vi "PrototypeV2_control.vi"() -> ()   [LabVIEW 2019]
uses:
  <vilib>/Instr/_visa.llb/VISA Configure Serial Port (Instr).vi
panel:
  out "CONV2":cluster{dbl, dbl, dbl}(graph)
  out "converter2 file":path
  out "controller file":path
  out "converter1 file":path
  in  "CONVERTER 2 PORT":refnum<visa-resource-name>="COM4"
  out "sync":bool
  in  "CONVERTER 2":bool
  in  "CONVERTER 1 PORT":refnum<visa-resource-name>="COM4"
  out "sync":bool
  in  "CONVERTER 1":bool
  out "CONV1":cluster{dbl, dbl, dbl}(graph)
  out "3.3V REG":cluster{dbl, dbl}(graph)
  out "5V REG":cluster{dbl, dbl}(graph)
  out "BUS":cluster{dbl, dbl, dbl}(graph)
  in  "project name":string
  in  "START":bool
  in  "CONTROLLER PORT":refnum<visa-resource-name>="COM4"
  out "sync":bool
  in  "CONTROLLER":bool
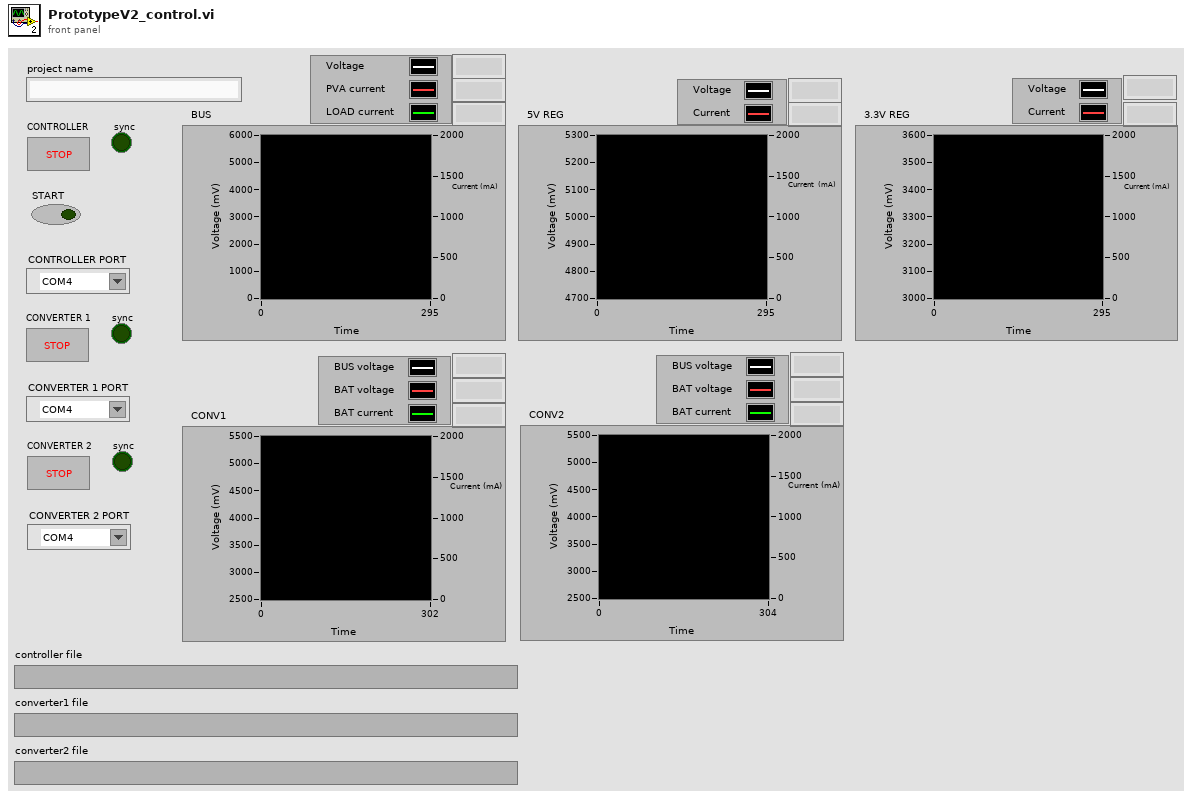
[diagram p1: front panel]
types:
  T1 = cluster{u16, u16, u16, u16, u16, u16, u16, u16, u16}
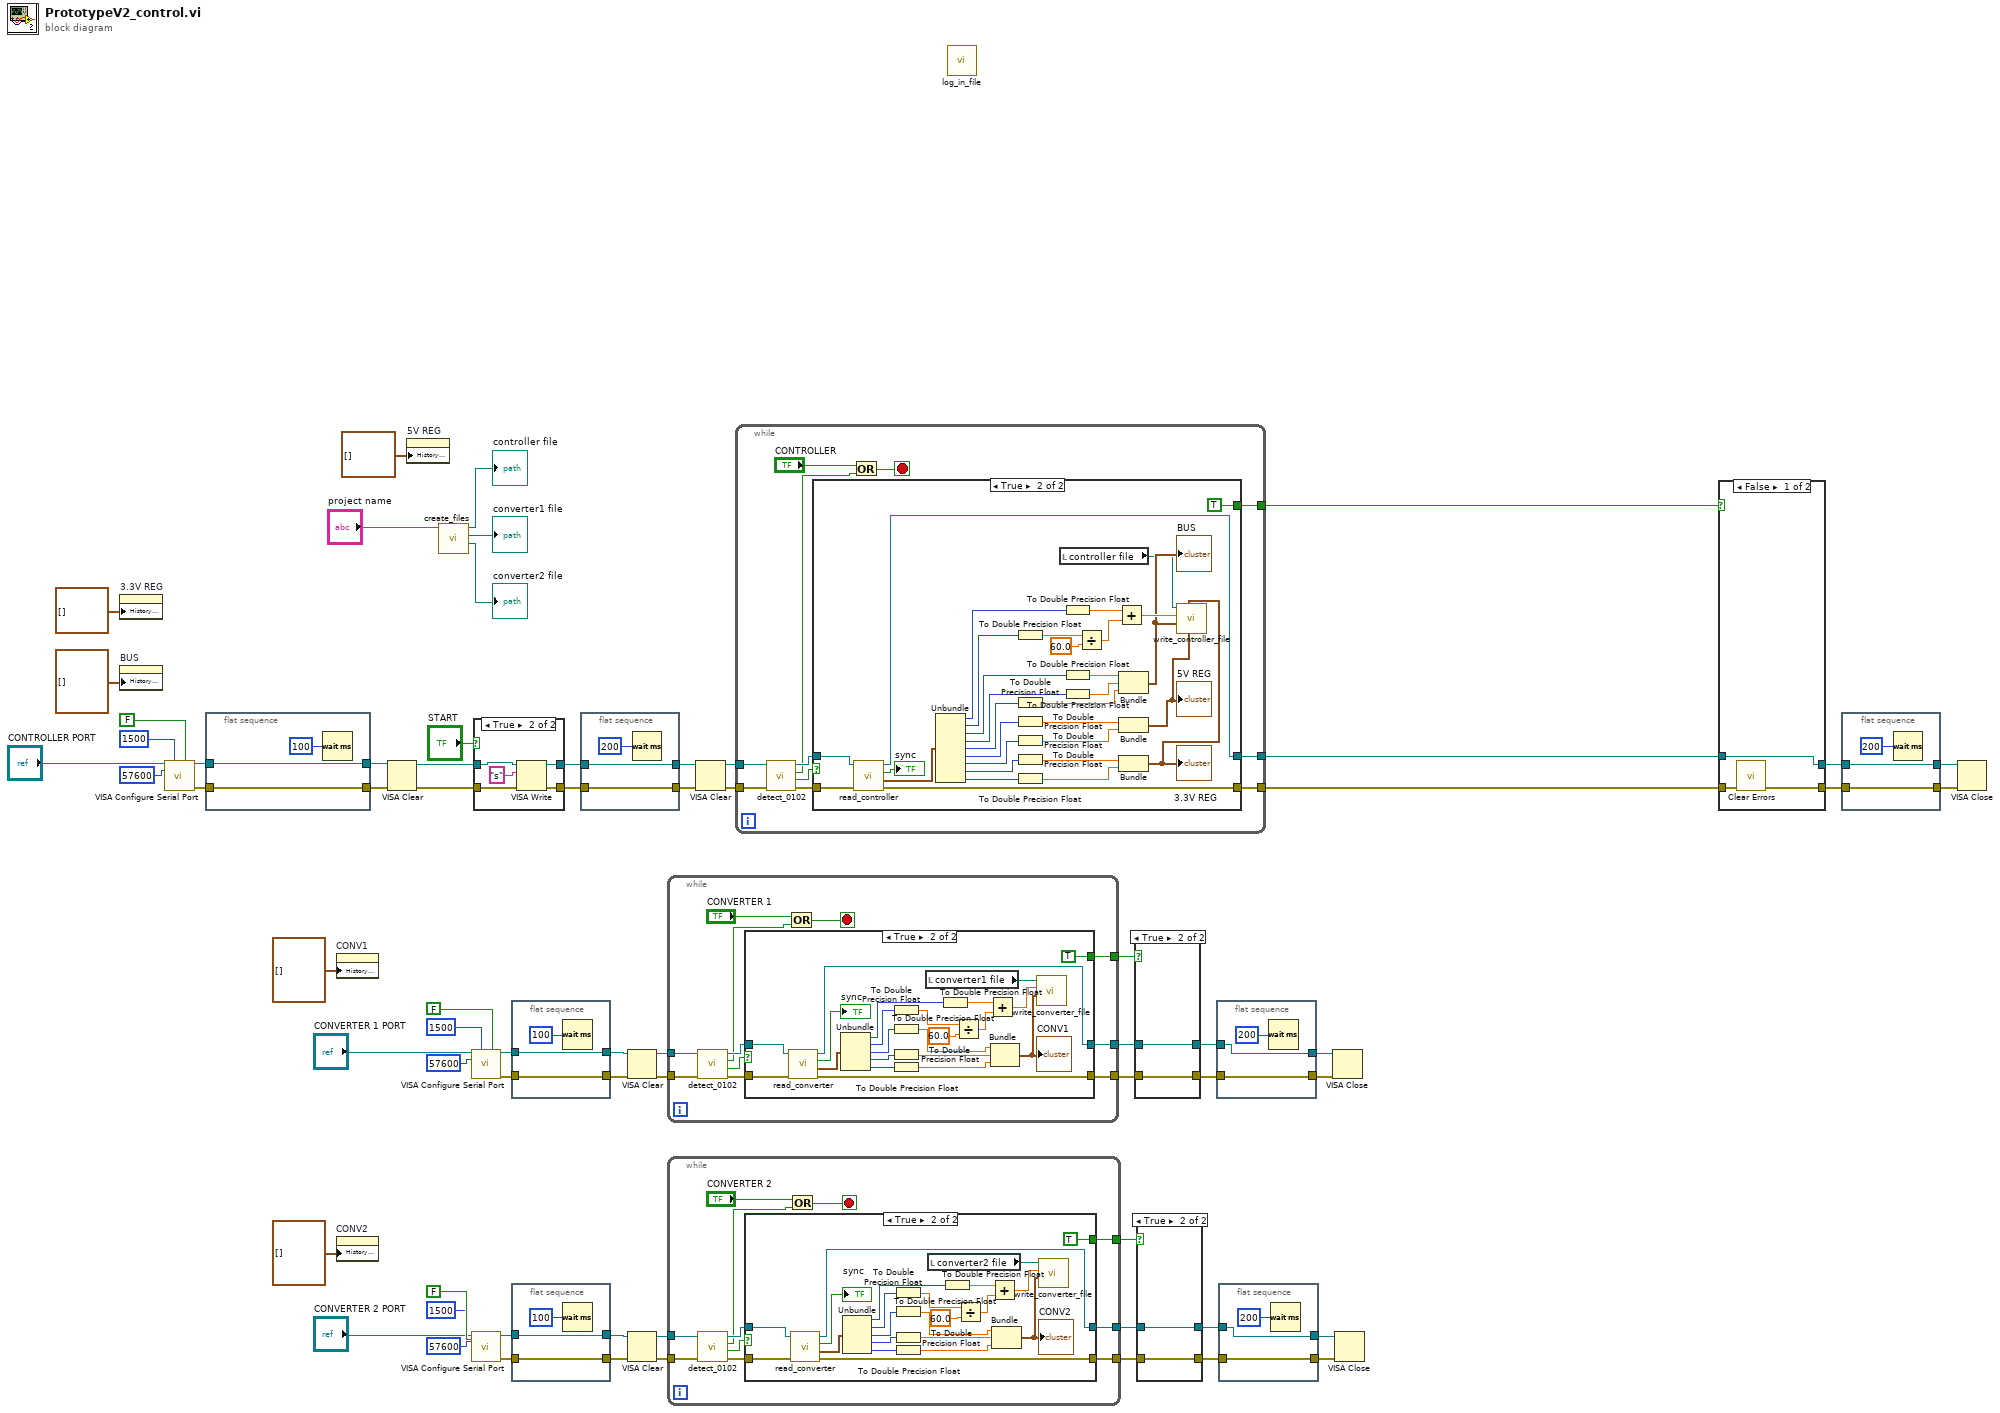
[diagram p0: block diagram]
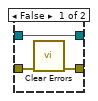
[diagram p2: hidden frame]
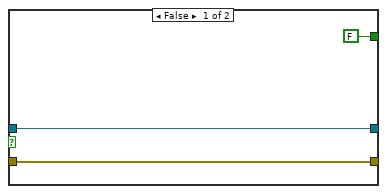
[diagram p3: hidden frame]
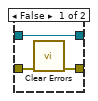
[diagram p4: hidden frame]
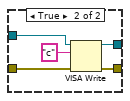
[diagram p5: hidden frame]
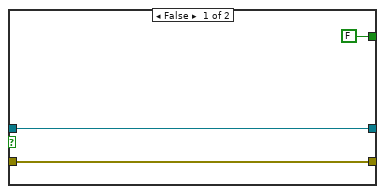
[diagram p6: hidden frame]
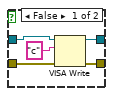
[diagram p7: hidden frame]
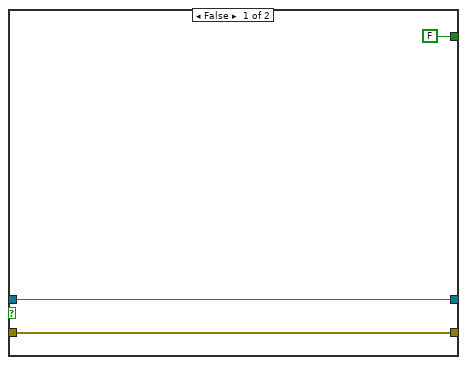
[diagram p8: hidden frame]
diagram:
  n1 = property on="3.3V REG" class="WFChart (strict)"("History Data"=cluster{dbl, dbl}[] []) -> ()  [unwired: 2 in, 2 out]
  n2 = property on="BUS" class="WFChart (strict)"("History Data"=cluster{dbl, dbl, dbl}[] []) -> ()  [unwired: 2 in, 2 out]
  n3 = call-poly "VISA Configure Serial Port"("VISA resource name"="CONTROLLER PORT", "timeout (10sec)"=u32 1500, "Enable Termination\nChar (T)"=FALSE ("Enable Termination\nChar (T)"), "baud rate (9600)"=u32 57600) -> ("VISA resource name out"=w64:refnum<visa-resource-name>, "error out"=w63:errorcluster)  [unwired: 10 in]
  n4 = flat-sequence {
    tunnel: w63 -> [w69]
    tunnel: [w69] -> w62
    tunnel: [w68] -> w61
    tunnel: w64 -> [w68]
    frame #0 {
      n5 = Wait (ms)(milliseconds to wait=u32 100) -> ()  [unwired: 1 out]
    }
  }
  n6 = property on="CONV1" class="WFChart (strict)"("History Data"=cluster{dbl, dbl, dbl}[] []) -> ()  [unwired: 2 in, 2 out]
  n7 = property on="CONV2" class="WFChart (strict)"("History Data"=cluster{dbl, dbl, dbl}[] []) -> ()  [unwired: 2 in, 2 out]
  n8 = VISA Clear(VISA resource name=w61, error in (no error)=w62) -> (VISA resource name out=w60:refnum<visa-resource-name>, error out=w59:errorcluster)
  n9 = property on="5V REG" class="WFChart (strict)"("History Data"=cluster{dbl, dbl}[] []) -> ()  [unwired: 2 in, 2 out]
  n10 = call "create_files.vi"("project name"="project name") -> ("converter2"=→"converter2 file":path, "converter1"=→"converter1 file":path, "controller"=→"controller file":path)  [unwired: 8 in]
  n11 = call-poly "VISA Configure Serial Port"("VISA resource name"="CONVERTER 1 PORT", "timeout (10sec)"=u32 1500, "Enable Termination\nChar (T)"=FALSE ("Enable Termination\nChar (T)"), "baud rate (9600)"=u32 57600) -> ("VISA resource name out"=w39:refnum<visa-resource-name>, "error out"=w38:errorcluster)  [unwired: 10 in]
  n12 = call-poly "VISA Configure Serial Port"("VISA resource name"="CONVERTER 2 PORT", "timeout (10sec)"=u32 1500, "Enable Termination\nChar (T)"=FALSE ("Enable Termination\nChar (T)"), "baud rate (9600)"=u32 57600) -> ("VISA resource name out"=w16:refnum<visa-resource-name>, "error out"=w15:errorcluster)  [unwired: 10 in]
  n13 = case shown="True" "START" {
    tunnel: w60 -> [w74 w80]
    tunnel: [w72 w79] -> w57
    tunnel: w59 -> [w73 w78]
    tunnel: [w71 w77] -> w56
    frame False {
      n14 = VISA Write(VISA resource name=w74, write buffer="c", error in (no error)=w73) -> (VISA resource name out=w72:refnum<visa-resource-name>, error out=w71:errorcluster)  [unwired: 1 out]
    }
    frame True {
      n15 = VISA Write(VISA resource name=w80, write buffer="s", error in (no error)=w78) -> (VISA resource name out=w79:refnum<visa-resource-name>, error out=w77:errorcluster)  [unwired: 1 out]
    }
  }
  n16 = flat-sequence {
    tunnel: w38 -> [w82]
    tunnel: [w82] -> w37
    tunnel: [w81] -> w36
    tunnel: w39 -> [w81]
    frame #0 {
      n17 = Wait (ms)(milliseconds to wait=u32 100) -> ()  [unwired: 1 out]
    }
  }
  n18 = flat-sequence {
    tunnel: w15 -> [w85]
    tunnel: [w85] -> w14
    tunnel: [w84] -> w13
    tunnel: w16 -> [w84]
    frame #0 {
      n19 = Wait (ms)(milliseconds to wait=u32 100) -> ()  [unwired: 1 out]
    }
  }
  n20 = flat-sequence {
    tunnel: w56 -> [w88]
    tunnel: [w88] -> w53
    tunnel: [w87] -> w55
    tunnel: w57 -> [w87]
    frame #0 {
      n21 = Wait (ms)(milliseconds to wait=u32 200) -> ()  [unwired: 1 out]
    }
  }
  n22 = VISA Clear(VISA resource name=w36, error in (no error)=w37) -> (VISA resource name out=w21:refnum<visa-resource-name>, error out=w20:errorcluster)
  n23 = VISA Clear(VISA resource name=w13, error in (no error)=w14) -> (VISA resource name out=w4:refnum<visa-resource-name>, error out=w3:errorcluster)
  n24 = while {
    tunnel: w20 -> [w94]
    tunnel: [w99] -> w27
    tunnel: [w100] -> w28
    tunnel: w21 -> [w95]
    tunnel: [w96] -> w26
    stop <- w97 stop-if-true
    n25 = call "detect_0102.vi"("error in (no error)"=w94, "VISA Refnum in"=w95) -> ("error out"=w92:errorcluster, "RECEIVED"=w90:bool, "NOT RECEIVED"=w91:bool, "VISA Refnum out"=w93:refnum<visa-resource-name>)  [unwired: 6 in]
    n26 = case shown="True" w90 {
      tunnel: w93 -> [w103 w112]
      tunnel: w92 -> [w102 w107]
      tunnel: [w103 w108] -> w100
      tunnel: [w102 w111] -> w99
      tunnel: [FALSE TRUE] -> w96
      frame False {
      }
      frame True {
        n27 = call "read_converter.vi"("error in (no error)"=w107, "VISA Refnum in"=w112) -> ("error out"=w111:errorcluster, "Types?"=w109:cluster{u16, u16, u16, u16, i16}, "sync"=→"sync":bool, "VISA Refnum out"=w108:refnum<visa-resource-name>)  [unwired: 6 in]
        n28 = Unbundle(w109) -> (w125:u16, w124:u16, w119:u16, w118:u16, w117:i16)
        n29 = To Double Precision Float(number=w124) -> (double precision float=w122:dbl)
        n30 = To Double Precision Float(number=w119) -> (double precision float=w116:dbl)
        n31 = To Double Precision Float(number=w118) -> (double precision float=w115:dbl)
        n32 = To Double Precision Float(number=w117) -> (double precision float=w114:dbl)
        n33 = local read "converter1 file"() -> (w105:path)
        n34 = To Double Precision Float(number=w125) -> (double precision float=w121:dbl)
        n35 = Divide(x=w122, y=60.0) -> (x/y=w120:dbl)
        n36 = Add(x=w121, y=w120) -> (x+y=w106:dbl)
        n37 = Bundle(w116, w115, w114) -> (w104:cluster{dbl, dbl, dbl})  [unwired: 1 in]
        "CONV1" <- w104
        n38 = call "write_converter_file.vi"("CONVERTER"=w104, "minutes"=w106, "converter file"=w105) -> ()  [unwired: 9 in]
      }
    }
    n39 = Or(x="CONVERTER 1", y=w91) -> (x .or. y?=w97:bool)
  }
  n40 = while {
    tunnel: w3 -> [w131]
    tunnel: [w135] -> w6
    tunnel: [w136] -> w7
    tunnel: w4 -> [w132]
    tunnel: [w133] -> w5
    stop <- w134 stop-if-true
    n41 = call "detect_0102.vi"("error in (no error)"=w131, "VISA Refnum in"=w132) -> ("error out"=w129:errorcluster, "RECEIVED"=w127:bool, "NOT RECEIVED"=w128:bool, "VISA Refnum out"=w130:refnum<visa-resource-name>)  [unwired: 6 in]
    n42 = case shown="True" w127 {
      tunnel: w130 -> [w139 w148]
      tunnel: w129 -> [w138 w144]
      tunnel: [w139 w145] -> w136
      tunnel: [w138 w147] -> w135
      tunnel: [FALSE TRUE] -> w133
      frame False {
      }
      frame True {
        n43 = call "read_converter.vi"("error in (no error)"=w144, "VISA Refnum in"=w148) -> ("error out"=w147:errorcluster, "Types?"=w146:cluster{u16, u16, u16, u16, i16}, "sync"=→"sync":bool, "VISA Refnum out"=w145:refnum<visa-resource-name>)  [unwired: 6 in]
        n44 = Unbundle(w146) -> (w161:u16, w160:u16, w155:u16, w154:u16, w153:i16)
        n45 = To Double Precision Float(number=w160) -> (double precision float=w158:dbl)
        n46 = To Double Precision Float(number=w155) -> (double precision float=w152:dbl)
        n47 = To Double Precision Float(number=w154) -> (double precision float=w151:dbl)
        n48 = To Double Precision Float(number=w153) -> (double precision float=w150:dbl)
        n49 = local read "converter2 file"() -> (w140:path)
        n50 = To Double Precision Float(number=w161) -> (double precision float=w157:dbl)
        n51 = Divide(x=w158, y=60.0) -> (x/y=w156:dbl)
        n52 = Add(x=w157, y=w156) -> (x+y=w141:dbl)
        n53 = Bundle(w152, w151, w150) -> (w142:cluster{dbl, dbl, dbl})  [unwired: 1 in]
        "CONV2" <- w142
        n54 = call "write_converter_file.vi"("CONVERTER"=w142, "minutes"=w141, "converter file"=w140) -> ()  [unwired: 9 in]
      }
    }
    n55 = Or(x="CONVERTER 2", y=w128) -> (x .or. y?=w134:bool)
  }
  n56 = VISA Clear(VISA resource name=w55, error in (no error)=w53) -> (VISA resource name out=w54:refnum<visa-resource-name>, error out=w52:errorcluster)
  n57 = while {
    tunnel: w52 -> [w170]
    tunnel: [w167] -> w50
    tunnel: [w168] -> w51
    tunnel: w54 -> [w169]
    tunnel: [w162] -> w34
    stop <- w165 stop-if-true
    n58 = call "detect_0102.vi"("error in (no error)"=w170, "VISA Refnum in"=w169) -> ("error out"=w171:errorcluster, "RECEIVED"=w163:bool, "NOT RECEIVED"=w164:bool, "VISA Refnum out"=w172:refnum<visa-resource-name>)  [unwired: 6 in]
    n59 = case shown="True" w163 {
      tunnel: w172 -> [w175 w207]
      tunnel: w171 -> [w174 w206]
      tunnel: [w175 w195] -> w168
      tunnel: [w174 w194] -> w167
      tunnel: [FALSE TRUE] -> w162
      frame False {
      }
      frame True {
        n60 = call "read_controller.vi"("error in (no error)"=w206, "VISA Refnum in"=w207) -> ("error out"=w194:errorcluster, "Type?"=w205:T1, "sync"=→"sync":bool, "VISA Refnum out"=w195:refnum<visa-resource-name>)  [unwired: 6 in]
        n61 = Unbundle(w205) -> (w204:u16, w203:u16, w198:u16, w197:u16, w196:u16, w193:u16, w192:u16, w191:u16, w190:u16)
        n62 = To Double Precision Float(number=w203) -> (double precision float=w201:dbl)
        n63 = To Double Precision Float(number=w196) -> (double precision float=w184:dbl)
        n64 = To Double Precision Float(number=w193) -> (double precision float=w189:dbl)
        n65 = To Double Precision Float(number=w192) -> (double precision float=w188:dbl)
        n66 = To Double Precision Float(number=w191) -> (double precision float=w187:dbl)
        n67 = To Double Precision Float(number=w190) -> (double precision float=w186:dbl)
        n68 = local read "controller file"() -> (w178:path)
        n69 = To Double Precision Float(number=w204) -> (double precision float=w200:dbl)
        n70 = To Double Precision Float(number=w198) -> (double precision float=w182:dbl)
        n71 = To Double Precision Float(number=w197) -> (double precision float=w183:dbl)
        n72 = Divide(x=w201, y=60.0) -> (x/y=w199:dbl)
        n73 = Add(x=w200, y=w199) -> (x+y=w180:dbl)
        n74 = Bundle(w182, w183, w184) -> (w179:cluster{dbl, dbl, dbl})  [unwired: 1 in]
        "BUS" <- w179
        n75 = Bundle(w189, w188) -> (w177:cluster{dbl, dbl})  [unwired: 1 in]
        "5V REG" <- w177
        n76 = Bundle(w187, w186) -> (w176:cluster{dbl, dbl})  [unwired: 1 in]
        "3.3V REG" <- w176
        n77 = call "write_controller_file.vi"("5V reg"=w177, "3.3V reg"=w176, "BUS"=w179, "minutes"=w180, "controller file"=w178) -> ()  [unwired: 7 in]
      }
    }
    n78 = Or(x="CONTROLLER", y=w164) -> (x .or. y?=w165:bool)
  }
  n79 = call "log_in_file.vi"() -> ()  [unwired: 7 in]
  n80 = case shown="True" w26 {
    tunnel: w28 -> [w210 w212]
    tunnel: w27 -> [w209 w211]
    tunnel: [w210 w212] -> w32
    tunnel: [w208 w211] -> w31
    frame False {
      n81 = call <vilib>:"Clear Errors.vi"("error in (no error)"=w209) -> ("error out"=w208:errorcluster)  [unwired: 5 in, 1 out]
    }
    frame True {
    }
  }
  n82 = case shown="True" w5 {
    tunnel: w7 -> [w215 w217]
    tunnel: w6 -> [w214 w216]
    tunnel: [w215 w217] -> w11
    tunnel: [w213 w216] -> w10
    frame False {
      n83 = call <vilib>:"Clear Errors.vi"("error in (no error)"=w214) -> ("error out"=w213:errorcluster)  [unwired: 5 in, 1 out]
    }
    frame True {
    }
  }
  n84 = flat-sequence {
    tunnel: w31 -> [w219]
    tunnel: [w219] -> w30
    tunnel: [w218] -> w29
    tunnel: w32 -> [w218]
    frame #0 {
      n85 = Wait (ms)(milliseconds to wait=u32 200) -> ()  [unwired: 1 out]
    }
  }
  n86 = flat-sequence {
    tunnel: w10 -> [w222]
    tunnel: [w222] -> w9
    tunnel: [w221] -> w8
    tunnel: w11 -> [w221]
    frame #0 {
      n87 = Wait (ms)(milliseconds to wait=u32 200) -> ()  [unwired: 1 out]
    }
  }
  n88 = VISA Close(VISA resource name=w29, error in (no error)=w30) -> ()  [unwired: 1 out]
  n89 = VISA Close(VISA resource name=w8, error in (no error)=w9) -> ()  [unwired: 1 out]
  n90 = case shown="False" w34 {
    tunnel: w51 -> [w226 w230]
    tunnel: w50 -> [w225 w229]
    tunnel: [w226 w228] -> w49
    tunnel: [w224 w227] -> w48
    frame False {
      n91 = call <vilib>:"Clear Errors.vi"("error in (no error)"=w225) -> ("error out"=w224:errorcluster)  [unwired: 5 in, 1 out]
    }
    frame True {
      n92 = VISA Write(VISA resource name=w230, write buffer="c", error in (no error)=w229) -> (VISA resource name out=w228:refnum<visa-resource-name>, error out=w227:errorcluster)  [unwired: 1 out]
    }
  }
  n93 = flat-sequence {
    tunnel: w48 -> [w233]
    tunnel: [w233] -> w47
    tunnel: [w232] -> w46
    tunnel: w49 -> [w232]
    frame #0 {
      n94 = Wait (ms)(milliseconds to wait=u32 200) -> ()  [unwired: 1 out]
    }
  }
  n95 = VISA Close(VISA resource name=w46, error in (no error)=w47) -> ()  [unwired: 1 out]
